vi "TCL Current Event File.vi"() -> (3 "current event file":path)   [LabVIEW 2010]
uses:
  TCL Global.vi
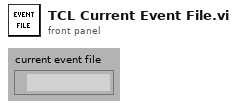
[diagram p1: front panel]
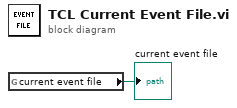
[diagram p0: block diagram]
diagram:
  n1 = global read "TCL Global.vi" "current event file"() -> (→"current event file":path)
